vi "Error_Handling_Test.vi"(11 "String":string) -> (3 "error out":errorcluster)   [LabVIEW 2024]
uses:
  Test Class 1/Test Class 1.lvclass
panel:
  out "specific class reference":refnum<class "Test Class 1.lvclass">
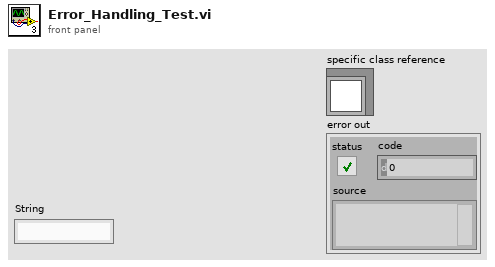
[diagram p1: front panel]
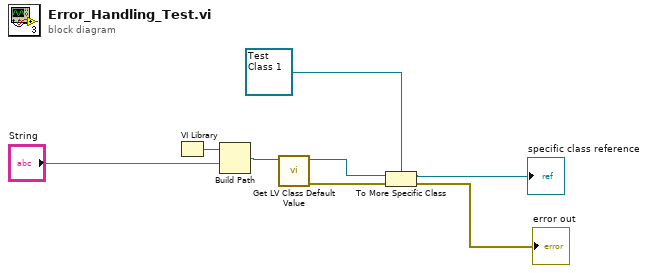
[diagram p0: block diagram]
diagram:
  n1 = VI Library() -> (path=w6:path)
  n2 = Build Path(base path=w6, name or relative path="String") -> (appended path=w5:path)
  n3 = call <vilib>:"Get LV Class Default Value.vi"("class path"=w5) -> ("error out"=w8:errorcluster, "object"=w7:refnum<class>)  [unwired: 9 in]
  n4 = To More Specific Class(target class=refnum<class "Test Class 1.lvclass"> refnum ("Test Class 1.lvclass"), reference=w7, error in=w8) -> (specific class reference=→"specific class reference":refnum<class "Test Class 1.lvclass">, error out=→"error out":errorcluster)
